vi "compute_slopes_on_image.vi"() -> ()   [LabVIEW 2018]
uses:
  Classes/HasoEngine/HasoEngine.lvclass
  Classes/Image/Image.lvclass
  Controls/SlopesEngineSetup.ctl
  Controls/Point2D.ctl
  Classes/HasoSlopes/HasoSlopes.lvclass
panel:
  out "Y Slopes":sgl[][](graph)
  in  "Image file name":string="Data\\data_image.himg"
  in  "Haso configuration file name":string="Data\\config_file_haso.dat"
  in  "Output file name":string="Data\\data_phase_computation_example.has"
  out "X Slopes":sgl[][](graph)
  out "error out":errorcluster
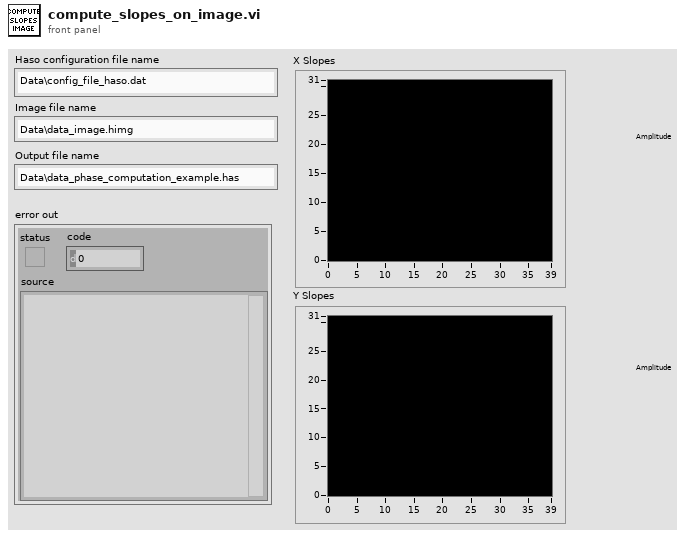
[diagram p1: front panel]
types:
  T1 = typedef "SlopesEngineSetup.ctl" = cluster{"Start sub-aperture":T2, "Pupil average":dbl, "AutoStartSub-aperture":bool}
  T2 = typedef "Point2D.ctl" = cluster{"X":u32, "Y":u32}
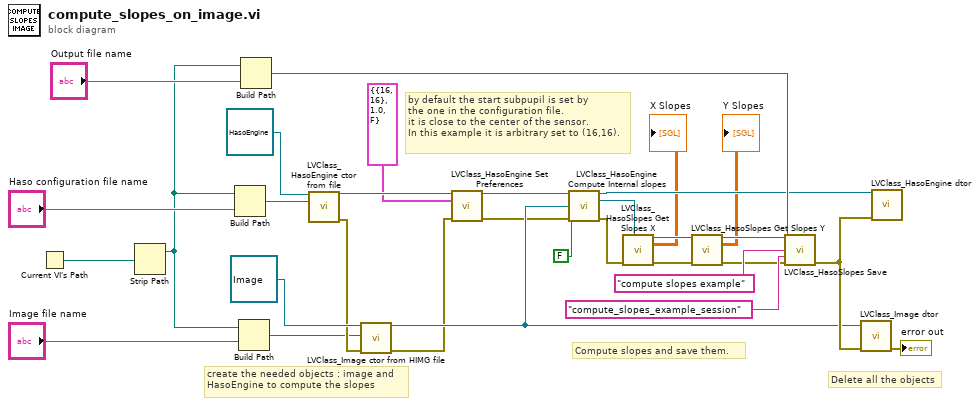
[diagram p0: block diagram]
diagram:
  # "Delete all the objects"
  # "Compute slopes and save them."
  # "by default the start subpupil is set by \nthe one in the configuration file. \nit is close to the center of the sensor.\nIn this example it is arbitrary set to (16,16)."
  # "create the needed objects : image and\nHasoEngine to compute the slopes"
  n1 = Current VI's Path() -> (path=w14:path)
  n2 = Strip Path(path=w14) -> (stripped path=w10:path)  [unwired: 1 out]
  n3 = Build Path(base path=w10, name or relative path="Haso configuration file name") -> (appended path=w9:path)
  n4 = Build Path(base path=w10, name or relative path="Image file name") -> (appended path=w11:path)
  n5 = Build Path(base path=w10, name or relative path="Output file name") -> (appended path=w24:path)
  n6 = call "LVClass_HasoEngine ctor from file.vi"("HasoEngine (const)"=refnum<class "HasoEngine.lvclass"> refnum ("HasoEngine in"), "Configuration file path"=w9) -> ("HasoEngine (new)"=w29:refnum<class "HasoEngine.lvclass">, "error out"=w18:errorcluster)  [unwired: 12 in]
  n7 = call "LVClass_Image ctor from HIMG file.vi"("Image (const)"=refnum<class "Image.lvclass"> refnum ("Image in"), "Path to image file"=w11, "error in (no error)"=w18) -> ("Image (new)"=w19:refnum<class "Image.lvclass">, "error out"=w17:errorcluster)  [unwired: 11 in]
  n8 = call "LVClass_HasoEngine Set Preferences.vi"("HasoEngine in"=w29, "Slopes_HasoEngine_Setup"=T1 {"Start sub-aperture"={"X"=16, "Y"=16}, "Pupil average"=1.0, "AutoStartSub-aperture"=FALSE}, "error in (no error)"=w17) -> ("HasoEngine out"=w27:refnum<class "HasoEngine.lvclass">, "error out"=w16:errorcluster)  [unwired: 11 in]
  n9 = call "LVClass_HasoEngine Compute Internal slopes.vi"("HasoEngine in"=w27, "Image.lvclass"=w19, "learn_from_trimmer"=FALSE, "error in (no error)"=w16) -> ("HasoEngine out"=w21:refnum<class "HasoEngine.lvclass">, "HasoSlopes (dup)"=w6:refnum<class "HasoSlopes.lvclass">, "error out"=w2:errorcluster)  [unwired: 7 in, 2 out]
  n10 = call "LVClass_HasoSlopes Get Slopes X.vi"("HasoSlopes in"=w6, "error in (no error)"=w2) -> ("HasoSlopes out"=w8:refnum<class "HasoSlopes.lvclass">, "Slopesx"=→"X Slopes":sgl[][], "error out"=w7:errorcluster)  [unwired: 11 in]
  n11 = call "LVClass_HasoSlopes Get Slopes Y.vi"("HasoSlopes in"=w8, "error in (no error)"=w7) -> ("HasoSlopes out"=w5:refnum<class "HasoSlopes.lvclass">, "Slopesy"=→"Y Slopes":sgl[][], "error out"=w1:errorcluster)  [unwired: 11 in]
  n12 = call "LVClass_HasoSlopes Save.vi"("HasoSlopes in"=w5, "path"=w24, "comments"="compute slopes example", "session"="compute_slopes_example_session", "error in (no error)"=w1) -> ("error out"=w20:errorcluster)  [unwired: 9 in, 1 out]
  n13 = call "LVClass_Image dtor.vi"("Image in"=w19, "error in (no error)"=w20) -> ("error out"=→"error out":errorcluster)  [unwired: 12 in, 1 out]
  n14 = call "LVClass_HasoEngine dtor.vi"("HasoEngine in"=w21, "error in (no error)"=w20) -> ()  [unwired: 12 in, 2 out]
